vi "Table Attributes Reset.vi"(11 "Table Refs":refnum<vi>[](array[refnum])) -> ()   [LabVIEW 2023, in "FPT Pulse Measurement UI.lvlib"]
uses:
  <vilib>/Utility/miscctls.llb/LVRowAndColumnTypeDef.ctl
  FPT Pulse Measurement UI.lvlib
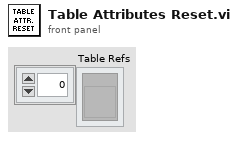
[diagram p1: front panel]
types:
  T1 = typedef "LVRowAndColumnTypeDef.ctl" = cluster{"Row":i32, "Column":i32}
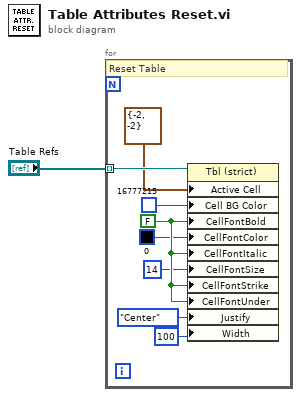
[diagram p0: block diagram]
diagram:
  n1 = for {
    tunnel: "Table Refs" -> [w9] mode=indexing
    w6 = FALSE ("Active Cell:Cell Font:Bold")
    # "Reset Table"
    n2 = property class="Tbl (strict)"(reference=w9, "Active Cell"=T1 {"Row"=-2, "Column"=-2} ("Active Cell:Active Cell"), "Cell BG Color"=u32 16777215 ("Active Cell:Cell Background Color"), "CellFontBold"=w6, "CellFontColor"=u32 0 ("Active Cell:Cell Font:Color"), "CellFontItalic"=w6, "CellFontSize"=u32 14 ("Active Cell:Cell Font:Size"), "CellFontStrike"=w6, "CellFontUnder"=w6, "Justify"=enum16{"Left", "Center", "Right"}."Center" ("Active Cell:Cell Justification"), "Width"=u32 100 ("Active Cell:Cell Size:Width")) -> ()  [unwired: 1 in, 2 out]
  }
